vi "BarcodeprintR567D.vi"(0 "二维图片 2":picture, 1 "字符串":string) -> ()   [LabVIEW 2020]
uses:
  Sources/Global_Variable/Global.vi
panel:
  out "法规号":string
  out "图号":string
  # "S"
  # "SW  VER: 00.01.00\nHW  VER: 0.0.1"
  # "201ABL\n4BS"
  # "CHN"
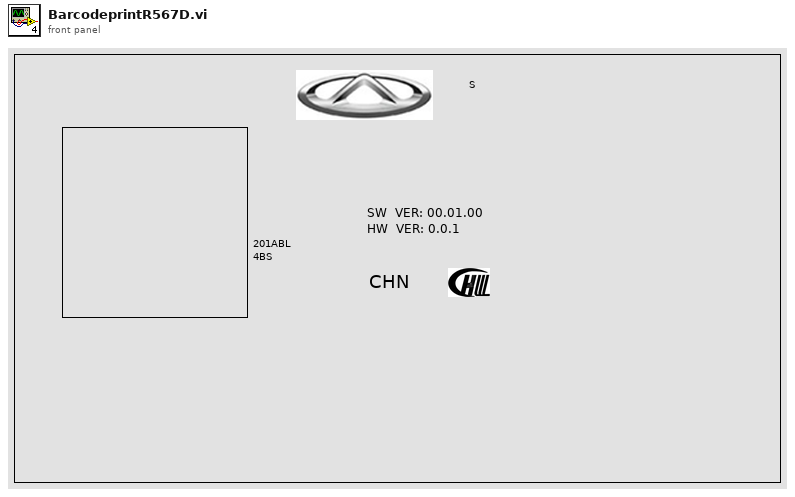
[diagram p1: front panel]
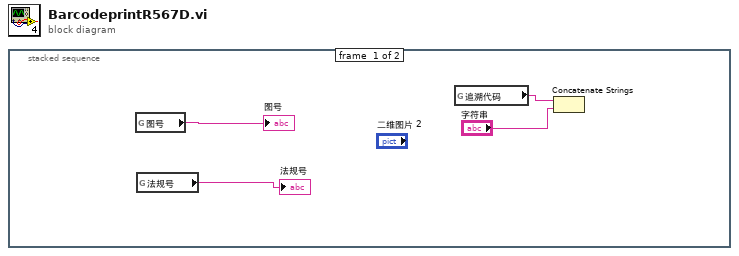
[diagram p0: block diagram]
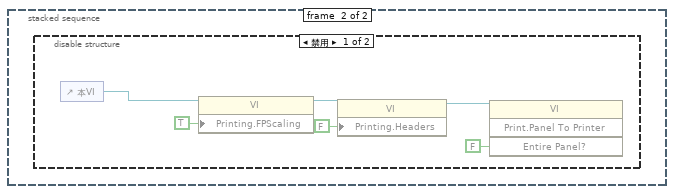
[diagram p2: hidden frame]
diagram:
  n1 = stacked-sequence {
    frame #0 {
      n2 = global read "Global.vi" "图号"() -> (→"图号":string)
      n3 = global read "Global.vi" "法规号"() -> (→"法规号":string)
      n4 = global read "Global.vi" "追溯代码"() -> (w2:string)
      n5 = Concatenate Strings(w2, "字符串") -> ()  [unwired: 1 out]
    }
    frame #1 {
      n6 = disable-structure shown="禁用" {
        frame Disabled {
          n7 = control-ref of="本VI"() -> (w10:refnum<vi>)
          n8 = property class="VI"(reference=w10, "Printing.FPScaling"=TRUE ("打印:前面板缩放？")) -> (reference out=w8:refnum<vi>)  [unwired: 1 in, 1 out]
          n9 = property class="VI"(reference=w8, "Printing.Headers"=FALSE ("打印:页眉？")) -> (reference out=w6:refnum<vi>)  [unwired: 1 in, 1 out]
          n10 = invoke class="VI" method="Print.Panel To Printer"(reference=w6, "Entire Panel?"=FALSE ("整个前面板？")) -> ()  [unwired: 2 in, 4 out]
        }
        frame Enabled {
        }
      }
    }
  }
